vi "NF87XX.reset.vi"(0 "i ref in":refnum<vi>, 5 "error in (no error)":errorcluster) -> (14 "i ref out":refnum<vi>, 19 "error out":errorcluster)   [LabVIEW 2014, in "NF87XX.lvlib"]
doc: "Resets the driver as well as the controller: This method has side effects on other drivers attached to the same controller. This method restores the previously saved parameters and enables the driver.\n\nauthor: Dietrich Beck\ndata: 26-JUL-2004\n\n\nLicense Agreement for this software:\n\nCopyright (C)\nGesellschaft für Schwerionenforschung, GSI\nPlanckstr. 1\n64291 Darmstadt\nGermany\n\nContact: D.Beck@gsi.de \n\nThis program is free software; you can redistribute it and/or modify it under the terms of the GNU General Public License as published by the Free Software Foundation; either version 2 of the license, or (at your option) any later version.\n\nThis program is distributed in the hope that it will be useful, but WITHOUT ANY WARRANTY; without even the implied warranty of MERCHANTABILITY or FITNESS FOR A PARTICULAR PURPOSE. See the GNU General License for more details (http://www.gnu.org).\n\nGesellschaft für Schwerionenforschung, GSI\nPlanckstr. 1, 64291 Darmstadt, Germany\nFor all questions and ideas contact: M.Richter@gsi.de, H.Brand@gsi.de or D.Beck@gsi.de.\nLast update: 17-JUN-2004"
uses:
  NF87XX.lvlib
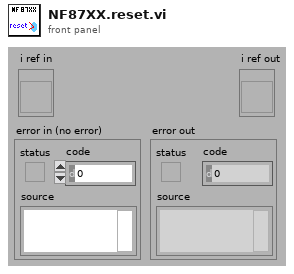
[diagram p1: front panel]
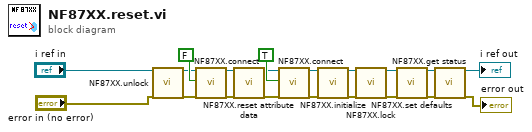
[diagram p0: block diagram]
diagram:
  n1 = call "NF87XX.unlock.vi"("i ref in"="i ref in", "error in (no error)"="error in (no error)") -> ("i ref out"=w17:refnum<vi>, "error out"=w16:errorcluster)  [unwired: 16 in]
  n2 = call "NF87XX.connect.vi"("i ref in"=w17, "Connect?"=FALSE ("Enable Driver"), "error in (no error)"=w16) -> ("i ref out"=w8:refnum<vi>, "error out"=w6:errorcluster)  [unwired: 15 in]
  n3 = call "NF87XX.reset attribute data.vi"("i ref in"=w8, "error in (no error)"=w6) -> ("i ref out"=w7:refnum<vi>, "error out"=w5:errorcluster)  [unwired: 16 in]
  n4 = call "NF87XX.connect.vi"("i ref in"=w7, "Connect?"=TRUE ("Open VISA?"), "error in (no error)"=w5) -> ("i ref out"=w12:refnum<vi>, "error out"=w13:errorcluster)  [unwired: 15 in]
  n5 = call "NF87XX.initialize.vi"("i ref in"=w12, "error in (no error)"=w13) -> ("i ref out"=w14:refnum<vi>, "error out"=w15:errorcluster)  [unwired: 16 in]
  n6 = call "NF87XX.lock.vi"("i ref in"=w14, "error in (no error)"=w15) -> ("i ref out"=w10:refnum<vi>, "error out"=w9:errorcluster)  [unwired: 16 in]
  n7 = call "NF87XX.set defaults.vi"("i ref in"=w10, "error in (no error)"=w9) -> ("i ref out"=w2:refnum<vi>, "error out"=w1:errorcluster)  [unwired: 16 in]
  n8 = call "NF87XX.get status.vi"("i ref in"=w2, "error in (no error)"=w1) -> ("i ref out"=→"i ref out":refnum<vi>, "error out"=→"error out":errorcluster)  [unwired: 15 in, 1 out]
